vi "afm_image_xyopenloop.vi"() -> ()   [LabVIEW 2015]
uses:
  controls/ControlParams_TF.ctl
  <vilib>/rvi/Emulation/niFpgaGetClockAttributes.vi
  <vilib>/rvi/Emulation/niFpgaSctlEmulationGetInTimedLoop.vi
  <vilib>/rvi/Emulation/niFpgaEmulationReportErrorSimple.vi
  <vilib>/rvi/interface/RandomDataEmulation/niFpgaRandomDataHandleErrors.vi
  <vilib>/rvi/eio/common/nirviEmuTemplateMethod_errors.vi
  <vilib>/rvi/Emulation/niFpgaCriticalErrorInLSC.vi
  <vilib>/rvi/DataTransferAndStorage/Container/XNode/niFpgaContainer.xnode
  <vilib>/rvi/interface/RandomDataEmulation/nirviRandomDataFpgaReadWriteTemplate.vi
  <vilib>/eio/EIONode/EIONode.xnode
panel:
  in  "Cluster":cluster{"TsTicks":u32, "force setpoint":sgl}
  in  "ControlParams":T1={"Umax "=0.0, "ymax"=0.0, "TsTicks"=0, "num"=[0.0, 0.0, 0.0, 0.0, 0.0, 0.0, 0.0, 0.0, 0.0], "den"=[0.0, 0.0, 0.0, 0.0, 0.0, 0.0, 0.0, 0.0, 0.0], "TF Order"=0, "num_ff"=[0.0, 0.0, 0.0, 0.0, 0.0, 0.0, 0.0, 0.0, 0.0], "den_ff"=[0.0, 0.0, 0.0, 0.0, 0.0, 0.0, 0.0, 0.0, 0.0], "TF_ff_order "=0, "ff_on"=FALSE}
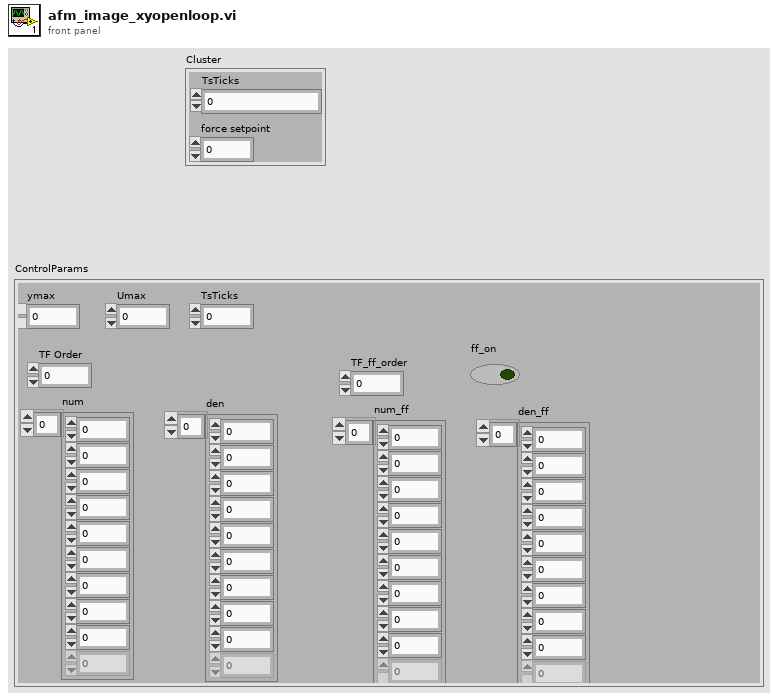
[diagram p1: front panel]
types:
  T1 = typedef "ControlParams_TF.ctl" = cluster{"Umax ":sgl, "ymax":sgl, "TsTicks":u32, "num":sgl[], "den":sgl[], "TF Order":u8, "num_ff":sgl[], "den_ff":sgl[], "TF_ff_order ":u8, "ff_on":bool}
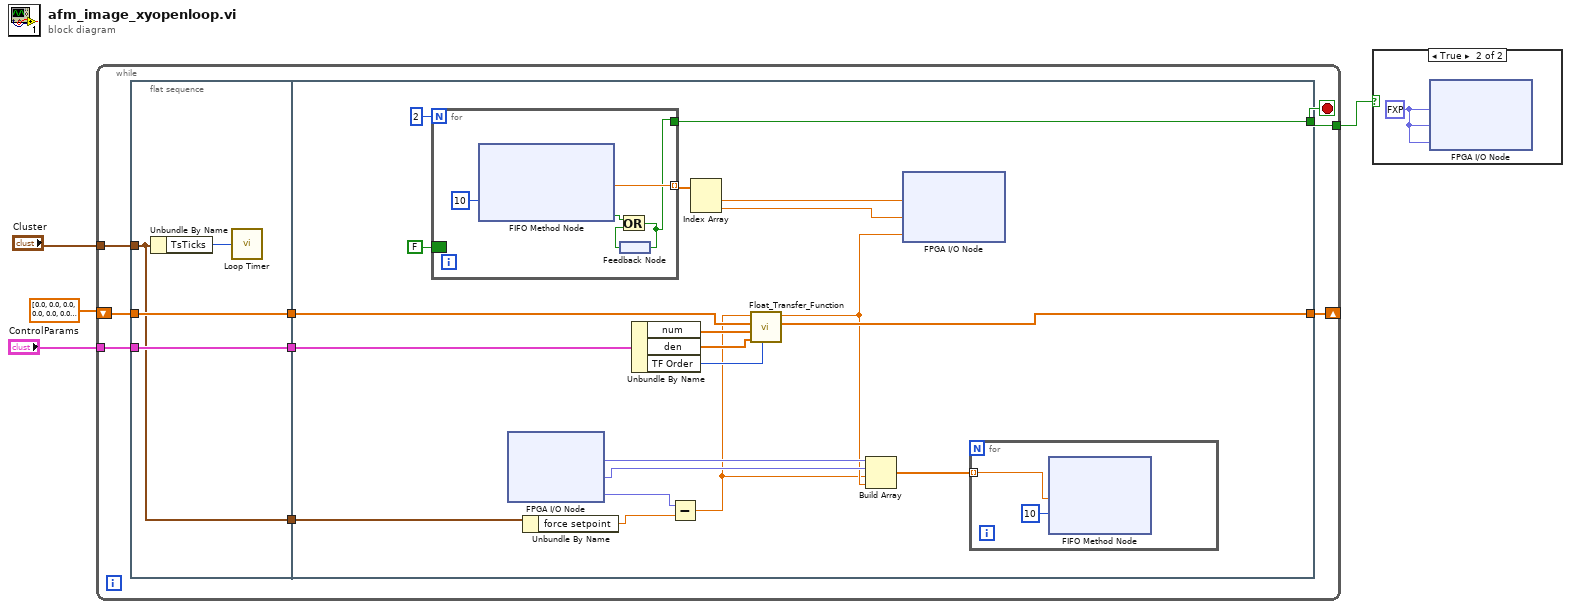
[diagram p0: block diagram]
diagram:
  n1 = while {
    tunnel: "ControlParams" -> [w12]
    shift-right: [w10] -> _
    shift-left: sgl[] [0.0, 0.0, 0.0, 0.0, 0.0, 0.0, 0.0, 0.0, 0.0] ("State Out") -> [w11]
    tunnel: [w7] -> w2
    tunnel: "Cluster" -> [w6]
    stop <- w7 stop-if-true
    n2 = flat-sequence {
      tunnel: w11 -> [w15]
      tunnel: w12 -> [w16]
      tunnel: [w16] -> w9
      tunnel: [w15] -> w8
      tunnel: w6 -> [w13]
      tunnel: [w13] -> w5
      tunnel: [w27] -> w10
      tunnel: w9 -> [w32]
      tunnel: w8 -> [w28]
      tunnel: [w21] -> w7
      tunnel: w5 -> [w20]
      frame #0 {
        n3 = Unbundle By Name(w13) -> ("TsTicks"=w14:u32)
        n4 = call "Loop Timer"("Count(Ticks)"=w14) -> ()  [unwired: 1 out]
      }
      frame #1 {
        n5 = for {
          N: 2 -> [_]
          tunnel: [w43] -> w35 mode=indexing
          border: FALSE -> [_]
          tunnel: [w39] -> w21
          n6 = xnode ("FIFO Method Node")("Timeout"=10) -> ("Element"=w43:sgl, "Timed Out?"=w41:bool)  [unwired: 1 in, 1 out]
          n7 = feedback #1() -> (w40:bool)
          n8 = Or(x=w41, y=w40) -> (x .or. y?=w39:bool)
          n9 = feedback-in #1(w39) -> ()
        }
        n10 = xnode "FPGA I/O Node"() -> ("Mod2/AI0"=w26:fxp<+/-,24,5>, "Mod2/AI1"=w25:fxp<+/-,24,5>, "Mod2/AI2"=w18:fxp<+/-,24,5>)  [unwired: 3 in, 3 out]
        n11 = Unbundle By Name(w20) -> ("force setpoint"=w19:sgl)
        n12 = Unbundle By Name(w32) -> ("num"=w31:sgl[], "den"=w30:sgl[], "TF Order"=w29:u8)
        n13 = Subtract(x=w18, y=w19) -> (x-y=w17:sgl)
        n14 = Index Array(array=w35) -> (element #1=w34:sgl, element #2=w33:sgl)  [unwired: 2 in]
        n15 = call "Float_Transfer_Function.vi"("TF Order"=w29, "Den"=w30, "Num"=w31, "State In"=w28, "Input"=w17) -> ("State Out"=w27:sgl[], "Output"=w24:sgl)  [unwired: 4 in]
        n16 = Build Array(w26, w25, w17, w24) -> (w23:sgl[])
        n17 = xnode "FPGA I/O Node"("Mod1/AO0"=w34, "Mod1/AO1"=w33, "Mod1/AO2"=w24) -> ()  [unwired: 3 in, 3 out]
        n18 = for {
          tunnel: w23 -> [w38] mode=indexing
          n19 = xnode ("FIFO Method Node")("Element"=w38, "Timeout"=10) -> ()  [unwired: 1 in, 2 out]
        }
      }
    }
  }
  n20 = case shown="True" w2 {
    frame False {
    }
    frame True {
      w44 = fxp<+/-,20,5> 0.0 ("Mod1/AO0")
      n21 = xnode "FPGA I/O Node"("Mod1/AO0"=w44, "Mod1/AO1"=w44, "Mod1/AO2"=w44) -> ()  [unwired: 3 in, 3 out]
    }
  }
